vi "VCI Set Filter.vi"(7 "pFilter":T1, 8 "error in (no error)":errorcluster, 9 "CANIndex":u32, 10 "DevIndex":u32, 11 "DevType":u32) -> (0 "error out":errorcluster, 3 "function return":u32)   [LabVIEW 2012, in "ControlCAN.lvlib"]
doc: "unsigned int WINAPI VCI_SetFilter(unsigned int DevType,unsigned int DevIndex,unsigned int CANIndex,PVCI_FILTER_CONFIG pFilter);"
uses:
  ControlCAN.lvlib
  Ginkgo_Driver.dll
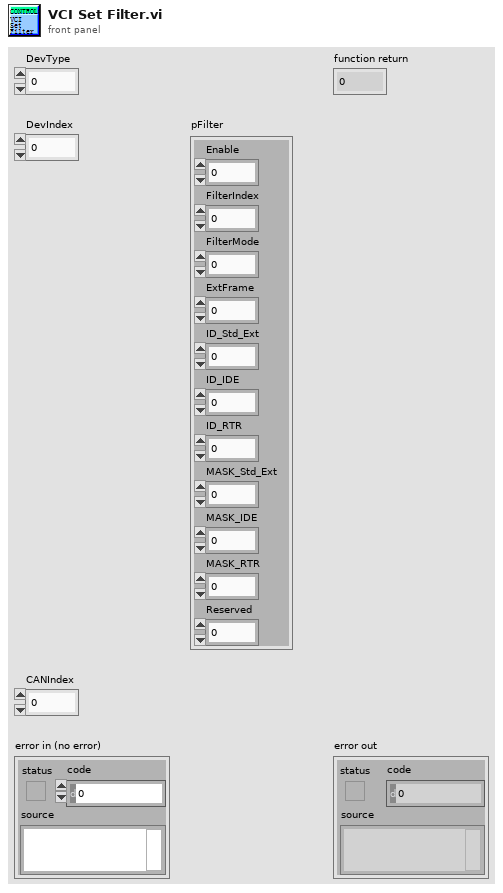
[diagram p1: front panel]
types:
  T1 = cluster{"Enable":u8, "FilterIndex":u8, "FilterMode":u8, "ExtFrame":u8, "ID_Std_Ext":u32, "ID_IDE":u32, "ID_RTR":u32, "MASK_Std_Ext":u32, "MASK_IDE":u32, "MASK_RTR":u32, "Reserved":u32}
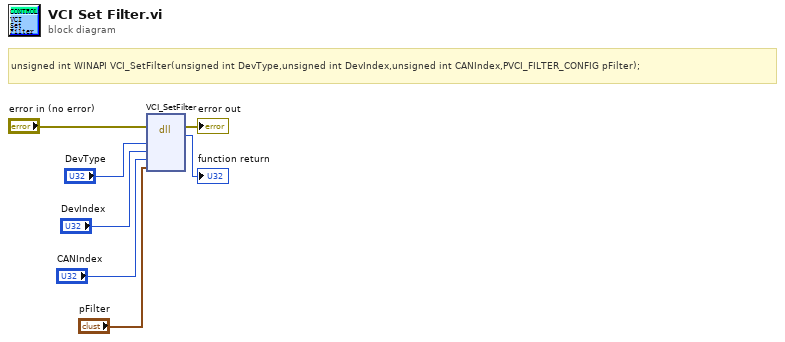
[diagram p0: block diagram]
diagram:
  # "unsigned int WINAPI VCI_SetFilter(unsigned int DevType,unsigned int DevIndex,unsigned int CANIndex,PVCI_FILTER_CONFIG pFilter);"
  n1 = dll-call lib="E:/Project/vt_ginkgo/truck/Ginkgo Driver/vs2010/Ginkgo_USB-I2C_API_v2.0.3.0/lib/labview_64bit/ControlCAN/Ginkgo_Driver.*" fn="VCI_SetFilter"(error in="error in (no error)", "DevType"="DevType", "DevIndex"="DevIndex", "CANIndex"="CANIndex", "pFilter"="pFilter") -> (error out=→"error out":errorcluster, →"function return":u32)  [unwired: 6 in, 1 out]
